vi "Create Sat Curves.vi"(10 "units":string(combo), 11 "fluid name":u16(ring)=17 items=["AIR.MIX", "AMARILLO.MIX", "EKOFISK.MIX", "GLFCOAST.MIX", "HIGHCO2.MIX", "HIGHN2.MIX", "NGSAMPLE.MIX", "R401A.MIX", "R401B.MIX", "R401C.MIX", "R402A.MIX", "R402B.MIX", "R403A.MIX", "R403B.MIX", "R405A.MIX", "R406A.MIX", "R407A.MIX", "R407B.MIX", "R407C.MIX", "R407D.MIX", "R407E.MIX", "R408A.MIX", "R409A.MIX", "R409B.MIX", "R410A.PPF", "R410B.MIX", "R411A.MIX", "R411B.MIX", "R412A.MIX", "R413A.MIX", "R414B.MIX", "R415A.MIX", "R415B.MIX", "R416A.MIX", "R417A.MIX", "R417B.MIX", "R417C.MIX", "R418A.MIX", "R419A.MIX", "R419B.MIX", "R420A.MIX", "R421A.MIX", "R421B.MIX", "R422A.MIX", "R422B.MIX", "R422C.MIX", "R422D.MIX", "R423A.MIX", "R424A.MIX", "R425A.MIX", "R426A.MIX", "R427A.MIX", "R428A.MIX", "R429A.MIX", "R430A.MIX", "R431A.MIX", "R432A.MIX", "R433A.MIX", "R433B.MIX", "R433C.MIX", "R434A.MIX", "R435A.MIX", "R436A.MIX", "R436B.MIX", "R437A.MIX", "R438A.MIX", "R439A.MIX", "R440A.MIX", "R441A.MIX", "R442A.MIX", "R443A.MIX", "R444A.MIX", "R444B.MIX", "R445A.MIX", "R446A.MIX", "R447A.MIX", "R448A.MIX", "R449A.MIX", "R449B.MIX", "R450A.MIX", "R451A.MIX", "R451B.MIX", "R452A.MIX", "R452B.MIX", "R452C.MIX", "R453A.MIX", "R454A.MIX", "R454B.MIX", "R454C.MIX", "R455A.MIX", "R456A.MIX", "R457A.MIX", "R459A.MIX", "R459B.MIX", "R460A.MIX", "R460B.MIX", "R500.MIX", "R501.MIX", "R502.MIX", "R503.MIX", "R504.MIX", "R507A.MIX", "R508A.MIX", "R508B.MIX", "R509A.MIX", "R510A.MIX", "R511A.MIX", "R512A.MIX", "R513A.MIX", "R513B.MIX", "R515A.MIX", "ammonia.fld", "butane.fld", "ethane.fld", "propane.fld", "R11.fld", "R113.fld", "R114.fld", "R115.fld", "R116.fld", "R12.fld", "R123.fld", "R124.fld", "R125.fld", "R13.fld", "R134a.fld", "R14.fld", "R141b.fld", "R142b.fld", "R143a.fld", "R152a.fld", "R161.fld", "R21.fld", "R218.fld", "R22.fld", "R227ea.fld", "R23.fld", "R236ea.fld", "R236fa.fld", "R245ca.fld", "R245fa.fld", "R32.fld", "R41.fld", "R1216.fld", "RC318.fld", "water.fld", "1butene.fld", "acetone.fld", "argon.fld", "benzene.fld", "c1cc6.fld", "c2butene.fld", "c3cc6.fld", "c4f10.fld", "c5f12.fld", "c11.fld", "c12.fld", "cf3i.fld", "CO.fld", "CO2.fld", "COS.fld", "cyclohex.fld", "cyclopen.fld", "cyclopro.fld", "D2.fld", "D2O.fld", "D4.fld", "D5.fld", "D6.fld", "decane.fld", "dee.fld", "dmc.fld", "dme.fld", "ebenzene.fld", "ethanol.fld", "ethylene.fld", "flourine.fld", "H2S.fld", "HCl.fld", "helium.fld", "heptane.fld", "hexane.fld", "hydrogen.fld", "ibutene.fld", "ihexane.fld", "ioctane.fld", "ipentane.fld", "isobutan.fld", "krypton.fld", "MD2M.fld", "MD3M.fld", "MD4M.fld", "MDM.fld", "methane.fld", "methanol.fld", "mlinolea.fld", "mlinolen.fld", "MM.fld", "moleate.fld", "mpalmita.fld", "mstearat.fld", "mxylene.fld", "N2O.fld", "neon.fld", "neopentn.fld", "NF3.fld", "nitrogen.fld", "nonane.fld", "novec649.fld", "octane.fld", "orthohyd.fld", "oxygen.fld", "parahyd.fld", "pentane.fld", "propylen.fld", "propyne.fld", "pxylene.fld", "R365MFC.fld", "R1233zd.fld", "R1234yf.fld", "R1234ze.fld", "RE143a.fld", "RE245cb2.fld", "RE245fa2.fld", "RE347mcc.fld", "sf6.fld", "SO2.fld", "T2butene.fld", "xenon.fld"]) -> (1 "pT":cluster{dbl[], dbl[]}, 2 "Ts":cluster{dbl[], dbl[]}, 3 "ph":cluster{dbl[], dbl[]})   [LabVIEW 2017]
panel:
  out "Critical Temperature (K) 2":dbl=72.58534253397343 format="%#_11g"
  out "Critical Pressure (kPa) 2":dbl
  out "Critical Temperature (K)":dbl=72.58534253397343 format="%#_11g"
  out "Critical Pressure (kPa)":dbl
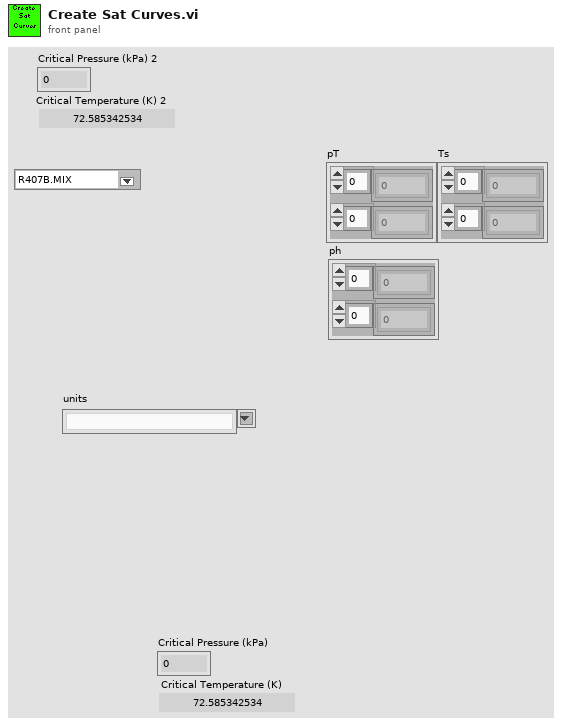
[diagram p1: front panel]
types:
  T1 = enum16{"0", "PS", "HS", "T", "P", "TP", "TH", "TS", "PH", "PQ", "TQ"}
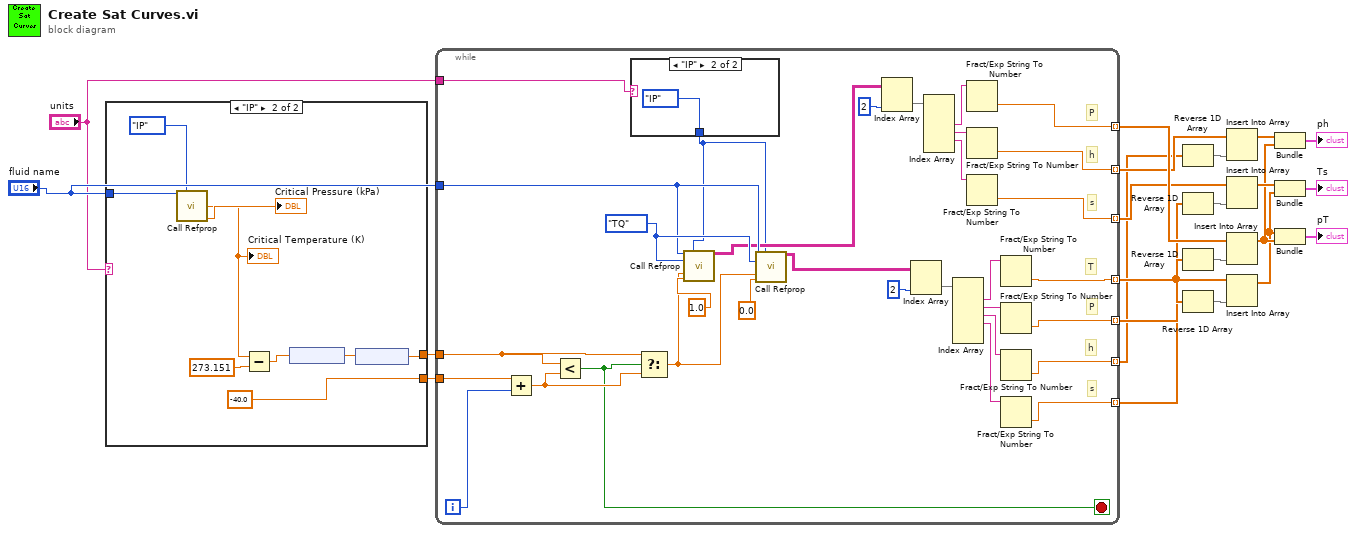
[diagram p0: block diagram]
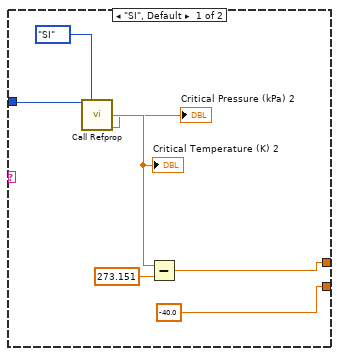
[diagram p2: hidden frame]
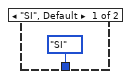
[diagram p3: hidden frame]
diagram:
  n1 = case shown="\"IP\"" "units" {
    tunnel: [-40.0 -40.0] -> w22
    tunnel: [w24 w32] -> w21
    tunnel: "fluid name" -> [w25 w35]
    frame "SI", Default {
      n2 = call "Call Refprop.vi"("fluid name"=w25, "units"=enum16{"SI", "IP"}."SI") -> ("Critical temperature (K)"=w29:dbl, "Critical Pressure (kPa)"=→"Critical Pressure (kPa) 2":dbl)  [unwired: 9 in, 3 out]
      "Critical Temperature (K) 2" <- w29
      n3 = Subtract(x=w29, y=273.151) -> (x-y=w24:dbl)
    }
    frame "IP" {
      n4 = call "Call Refprop.vi"("fluid name"=w35, "units"=enum16{"SI", "IP"}."IP") -> ("Critical temperature (K)"=w33:dbl, "Critical Pressure (kPa)"=→"Critical Pressure (kPa)":dbl)  [unwired: 9 in, 3 out]
      "Critical Temperature (K)" <- w33
      n5 = Subtract(x=w33, y=273.151) -> (x-y=w31:dbl)
      n6 = node(w31) -> (w30:dbl[unit])
      n7 = node(w30) -> (w32:dbl)
    }
  }
  n8 = while {
    tunnel: w22 -> [w70]
    tunnel: w21 -> [w68]
    tunnel: "fluid name" -> [w64]
    tunnel: [w56] -> w15 mode=indexing
    tunnel: [w54] -> w10 mode=indexing
    tunnel: [w52] -> w13 mode=indexing
    tunnel: [w50] -> w19 mode=indexing
    tunnel: [w45] -> w17 mode=indexing
    tunnel: [w43] -> w11 mode=indexing
    tunnel: [w41] -> w14 mode=indexing
    tunnel: "units" -> [w39]
    i -> [w69]
    stop <- w63 stop-if-true
    w65 = T1."TQ" ("InpCode")
    # "s"
    # "h"
    # "P"
    # "s"
    # "h"
    # "P"
    # "T"
    n9 = Add(x=w70, y=w69) -> (x+y=w67:dbl)
    n10 = Less?(x=w68, y=w67) -> (x < y?=w63:bool)
    n11 = case shown="\"IP\"" w39 {
      tunnel: [enum16{"SI", "IP"}."SI" ("units") enum16{"SI", "IP"}."IP" ("units")] -> w40
      frame "SI", Default {
      }
      frame "IP" {
      }
    }
    n12 = Select(t=w68, s=w63, f=w67) -> (s? t:f=w62:dbl)
    n13 = call "Call Refprop.vi"("fluid name"=w64, "units"=w40, "InpCode"=w65, "output_1"=w62, "output_2"=1.0) -> ("data"=w49:string[][])  [unwired: 6 in, 4 out]
    n14 = call "Call Refprop.vi"("fluid name"=w64, "units"=w40, "InpCode"=w65, "output_1"=w62, "output_2"=0.0) -> ("data"=w60:string[][])  [unwired: 6 in, 4 out]
    n15 = Index Array(array=w49, index (col)=2 ("disabled index (col)")) -> (element=w47:string[])  [unwired: 1 in]
    n16 = Index Array(array=w60, index (col)=2 ("disabled index (col)")) -> (element=w58:string[])  [unwired: 1 in]
    n17 = Index Array(array=w47) -> (element #2=w46:string, element #3=w44:string, element #4=w42:string)  [unwired: 5 in, 2 out]
    n18 = Index Array(array=w58) -> (element #1=w51:string, element #2=w57:string, element #3=w55:string, element #4=w53:string)  [unwired: 6 in, 2 out]
    n19 = Fract/Exp String To Number(string=w46) -> (number=w45:dbl)  [unwired: 3 in, 1 out]
    n20 = Fract/Exp String To Number(string=w44) -> (number=w43:dbl)  [unwired: 3 in, 1 out]
    n21 = Fract/Exp String To Number(string=w42) -> (number=w41:dbl)  [unwired: 3 in, 1 out]
    n22 = Fract/Exp String To Number(string=w51) -> (number=w50:dbl)  [unwired: 3 in, 1 out]
    n23 = Fract/Exp String To Number(string=w57) -> (number=w56:dbl)  [unwired: 3 in, 1 out]
    n24 = Fract/Exp String To Number(string=w55) -> (number=w54:dbl)  [unwired: 3 in, 1 out]
    n25 = Fract/Exp String To Number(string=w53) -> (number=w52:dbl)  [unwired: 3 in, 1 out]
  }
  n26 = Reverse 1D Array(array=w10) -> (reversed array=w9:dbl[])
  n27 = Reverse 1D Array(array=w13) -> (reversed array=w12:dbl[])
  n28 = Reverse 1D Array(array=w15) -> (reversed array=w16:dbl[])
  n29 = Reverse 1D Array(array=w19) -> (reversed array=w18:dbl[])
  n30 = Insert Into Array(array=w11, new element=w9) -> (w7:dbl[])  [unwired: 1 in]
  n31 = Insert Into Array(array=w14, new element=w12) -> (w8:dbl[])  [unwired: 1 in]
  n32 = Insert Into Array(array=w17, new element=w16) -> (w6:dbl[])  [unwired: 1 in]
  n33 = Insert Into Array(array=w19, new element=w18) -> (w5:dbl[])  [unwired: 1 in]
  n34 = Bundle(w7, w6) -> (→"ph":cluster{dbl[], dbl[]})  [unwired: 1 in]
  n35 = Bundle(w8, w5) -> (→"Ts":cluster{dbl[], dbl[]})  [unwired: 1 in]
  n36 = Bundle(w5, w6) -> (→"pT":cluster{dbl[], dbl[]})  [unwired: 1 in]
